vi "Configure Level Filter.vi"(8 "error in (no error)":errorcluster, 9 "Lowpass Filter (0: lpFsdiv2)":i32(ring) items=["lpFsdiv2", "lpHzAES20k", "lpHzAES40k", "lpHzAES80k"], 10 "Highpass Filter (0: hpDC)":i32(ring) items=["hpDC", "hpHz22", "hpHz100", "hpHz400", "hpSharp400"], 11 "VISA resource name":refnum<visa-resource-name>) -> (0 "error out":errorcluster, 3 "VISA resource name out":refnum<visa-resource-name>)   [LabVIEW 2014, in "Stanford Research SR1.lvlib"]
doc: "Configures the attributes for the Level Filter."
uses:
  Stanford Research SR1.lvlib
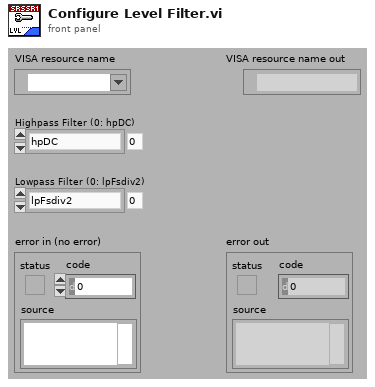
[diagram p1: front panel]
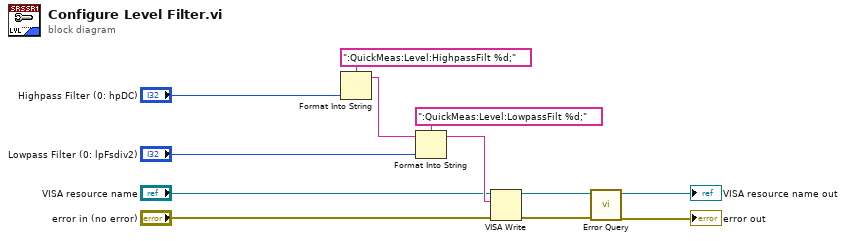
[diagram p0: block diagram]
diagram:
  n1 = Format Into String(format string=":QuickMeas:Level:HighpassFilt %d;", "Highpass Filter (0: hpDC)") -> (resulting string=w10:string)  [unwired: 2 in, 1 out]
  n2 = Format Into String(format string=":QuickMeas:Level:LowpassFilt %d;", initial string=w10, "Lowpass Filter (0: lpFsdiv2)") -> (resulting string=w7:string)  [unwired: 1 in, 1 out]
  n3 = VISA Write(VISA resource name="VISA resource name", write buffer=w7, error in (no error)="error in (no error)") -> (VISA resource name out=w4:refnum<visa-resource-name>, error out=w3:errorcluster)  [unwired: 1 out]
  n4 = call "Error Query.vi"("error in (no error)"=w3, "VISA resource name"=w4) -> ("error out"=→"error out":errorcluster, "VISA resource name out"=→"VISA resource name out":refnum<visa-resource-name>)  [unwired: 6 in, 2 out]
